vi "Tests - XWPF Writer.vi"(8 "error in (no error)":errorcluster) -> (0 "error out":errorcluster)   [LabVIEW 2017]
uses:
  src/Styles/Title/Title.lvclass
  C:/Users/Neo/Desktop/Dev_Tools_BR/LabVIEW_NPOI/src/Styles/Style/Style.lvclass
  src/Styles/Heading 1/Heading 1.lvclass
  C:/Users/Neo/Desktop/Dev_Tools_BR/LabVIEW_NPOI/src/Styles/Heading/Heading.lvclass
  src/Styles/Heading 2/Heading 2.lvclass
  src/Styles/Heading 3/Heading 3.lvclass
  src/Styles/Heading/Heading.lvclass
  <vilib>/addons/_JKI Toolkits/Caraya/classes/Assert/Assert Not Error.vi
  <vilib>/addons/_JKI Toolkits/Caraya/classes/Assert/Assert True.vi
  src/LabVIEW NPOI/xwpfWriter/xwpfWriter.lvclass
  <vilib>/addons/_JKI Toolkits/Caraya/classes/Test/Test.lvclass
  <vilib>/addons/_JKI Toolkits/Caraya/classes/Assert/Assert.lvclass
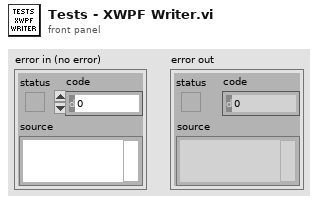
[diagram p1: front panel]
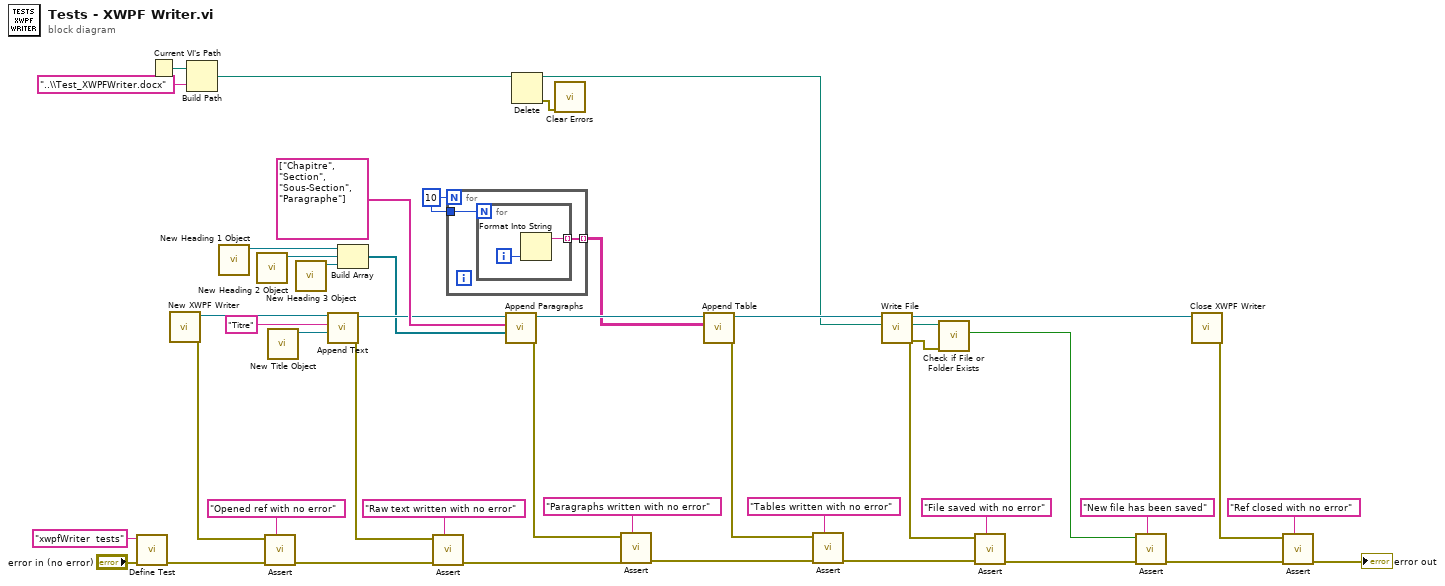
[diagram p0: block diagram]
diagram:
  w31 = 10
  n1 = call <vilib>:"Define Test.vi"("error in (no error)"="error in (no error)", "Label (VI Title)"="xwpfWriter  tests") -> ("error out"=w27:errorcluster)  [unwired: 9 in]
  n2 = Current VI's Path() -> (path=w16:path)
  n3 = call "New XWPF Writer.vi"() -> ("error out"=w15:errorcluster, "xwpfWriter out"=w43:refnum<class "xwpfWriter.lvclass">)  [unwired: 10 in]
  n4 = Build Path(base path=w16, name or relative path="..\\Test_XWPFWriter.docx" ("string")) -> (appended path=w4:path)
  n5 = call "New Heading 1 Object.vi"() -> ("Heading 1 out"=w37:refnum<class "Heading 1.lvclass">)  [unwired: 10 in, 1 out]
  n6 = call "New Heading 2 Object.vi"() -> ("Heading 2 out"=w36:refnum<class "Heading 2.lvclass">)  [unwired: 10 in, 1 out]
  n7 = call-poly <vilib>:"Assert.vi"("Label"="Opened ref with no error", "error in (no error)"=w27, "Not Error?"=w15) -> ("error out"=w21:errorcluster)  [unwired: 8 in]
  n8 = call "New Title Object.vi"() -> ("Title out"=w38:refnum<class "Title.lvclass">)  [unwired: 10 in, 1 out]
  n9 = call "New Heading 3 Object.vi"() -> ("Heading 3 out"=w35:refnum<class "Heading 3.lvclass">)  [unwired: 10 in, 1 out]
  n10 = call "Append Text.vi"("Style"=w38, "Text"="Titre", "xwpfWriter in"=w43) -> ("error out"=w14:errorcluster, "xwpfWriter out"=w39:refnum<class "xwpfWriter.lvclass">)  [unwired: 7 in]
  n11 = Build Array(w37, w36, w35) -> (w34:refnum<class "Heading.lvclass">[])
  n12 = call-poly <vilib>:"Assert.vi"("Label"="Raw text written with no error", "error in (no error)"=w21, "Not Error?"=w14) -> ("error out"=w20:errorcluster)  [unwired: 8 in]
  n13 = for {
    N: w31 -> [_]
    tunnel: [w45] -> w30 mode=indexing
    tunnel: w31 -> [w44]
    n14 = for {
      N: w44 -> [_]
      tunnel: [w46] -> w45 mode=indexing
      i -> [w47]
      n15 = Format Into String(w47) -> (resulting string=w46:string)  [unwired: 3 in, 1 out]
    }
  }
  n16 = call "Append Paragraphs.vi"("Styles"=w34, "Paragraphs"=string[] ["Chapitre", "Section", "Sous-Section", "Paragraphe"], "xwpfWriter in"=w39) -> ("error out"=w13:errorcluster, "xwpfWriter out"=w33:refnum<class "xwpfWriter.lvclass">)  [unwired: 7 in]
  n17 = Delete(path (use dialog)=w4) -> (deleted path=w3:path, error out=w2:errorcluster)  [unwired: 4 in, 1 out]
  n18 = call <vilib>:"Clear Errors.vi"("error in (no error)"=w2) -> ()  [unwired: 5 in, 2 out]
  n19 = call-poly <vilib>:"Assert.vi"("Label"="Paragraphs written with no error", "error in (no error)"=w20, "Not Error?"=w13) -> ("error out"=w19:errorcluster)  [unwired: 8 in]
  n20 = call "Append Table.vi"("Table"=w30, "xwpfWriter in"=w33) -> ("error out"=w12:errorcluster, "xwpfWriter out"=w32:refnum<class "xwpfWriter.lvclass">)  [unwired: 8 in]
  n21 = call-poly <vilib>:"Assert.vi"("Label"="Tables written with no error", "error in (no error)"=w19, "Not Error?"=w12) -> ("error out"=w18:errorcluster)  [unwired: 8 in]
  n22 = call "Write File.vi"("path"=w3, "xwpfWriter in"=w32) -> ("error out"=w1:errorcluster, "xwpfWriter out"=w42:refnum<class "xwpfWriter.lvclass">)  [unwired: 8 in]
  n23 = call <vilib>:"Check if File or Folder Exists.vi"("error in (no error)"=w1, "path"=w3) -> ("file or folder exists?"=w6:bool)  [unwired: 7 in, 2 out]
  n24 = call-poly <vilib>:"Assert.vi"("Label"="File saved with no error", "error in (no error)"=w18, "Not Error?"=w1) -> ("error out"=w7:errorcluster)  [unwired: 8 in]
  n25 = call-poly <vilib>:"Assert.vi"("Label"="New file has been saved", "error in (no error)"=w7, "True?"=w6) -> ("error out"=w5:errorcluster)  [unwired: 8 in]
  n26 = call "Close XWPF Writer.vi"("xwpfWriter in"=w42) -> ("error out"=w9:errorcluster)  [unwired: 9 in, 1 out]
  n27 = call-poly <vilib>:"Assert.vi"("Label"="Ref closed with no error", "error in (no error)"=w5, "Not Error?"=w9) -> ("error out"=→"error out":errorcluster)  [unwired: 8 in]
